vi "HistoryList.vi"(7 "Module Name":string="Module") -> ()   [LabVIEW 2017, in "DebugConsole.lvlib"]
uses:
  DebugConsole.lvlib
  508e9bfe-6490-4ffa-b47f-27ea34313f76.vi
  089f3262-7a84-4d39-9c60-bc06a6c67321.vi
  a9ada03b-0598-4474-9d19-b17bf33f6bd0.vi
  <vilib>/addons/_JKI Toolkits/State Machine/_JKI_lib_State_Machine.llb/Parse State Queue__JKI_lib_State_Machine.vi
  AdvanceAPI/CSM - Keywords.vi
  _csmlite/_Engine.vi
  _csmlite/_PassAllowedMessage - Mapping.vi
  _Polymophic/CSM - Replace Marks in Messages.vi
  <vilib>/Utility/Data Type/Get Type Information.vi
  _csmHelper/lvcsmFile/lvcsm File Path.vi
  <vilib>/Utility/config.llb/Open Config Data.vi
  <vilib>/Utility/config.llb/Write Key.vi
  <vilib>/Utility/config.llb/Write Key (Boolean).vi
  <vilib>/Utility/Data Type/Get Array Information.vi
  <vilib>/Utility/config.llb/Get Key Names.vi
  <vilib>/Utility/config.llb/Remove Key.vi
  <vilib>/Utility/config.llb/Write Key (String).vi
  _csmHelper/lvcsmFile/Path to lvcsm String.vi
  <vilib>/Utility/config.llb/Write Key (I32).vi
  <vilib>/Utility/config.llb/Write Key (Double).vi
  <vilib>/Utility/config.llb/Close Config Data.vi
  _Polymophic/Add State(s) to Queue By BOOL(Element).vi
  <vilib>/Utility/config.llb/Read Key.vi
  <vilib>/Utility/config.llb/Read Key (Boolean).vi
  <vilib>/Utility/config.llb/Read Key (String).vi
  _csmHelper/lvcsmFile/lvcsm String to Path.vi
  <vilib>/Utility/config.llb/Read Key (I32).vi
  <vilib>/Utility/config.llb/Read Key (Double).vi
  _csmHelper/lvcsmFile/_Array of VData to VCluster.vi
  _csmlite/_csmlite.lvlib
  Communicable State Machine.lvlib
  _Shared/CSM Shared.lvlib
panel:
  in  "History":i32(listbox)
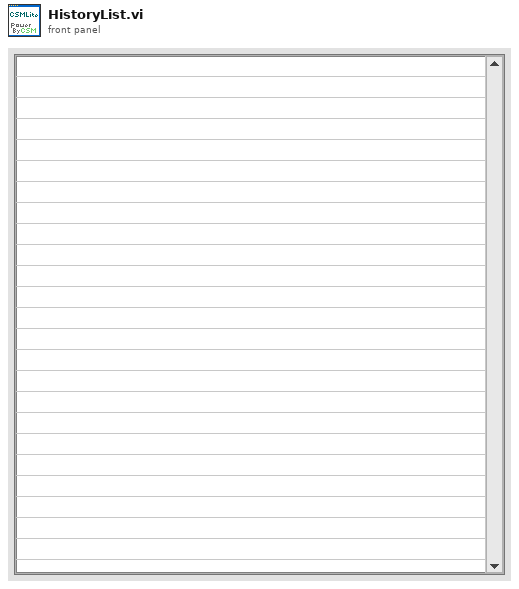
[diagram p1: front panel]
types:
  T1 = enum32{"Invalid", "Standard", "Closed", "Hidden", "Minimized", "Maximized"}
  T2 = enum32{"invalid app kind", "Development System", "Run Time System", "Student Edition", "Embedded LabVIEW", "Evaluation", "Custom"}
  T3 = cluster{"History Length":i32, "History":string[]}
  T4 = typedef "LVPoint32TypeDef.ctl" = cluster{"Horizontal":i32, "Vertical":i32}
  T5 = cluster{"Core":cluster{"Current VI Reference":refnum<vi>, "Close Panel on Exit?":bool}, "History Length":i32}
  T6 = cluster{"Current VI Reference":refnum<vi>, "Close Panel on Exit?":bool}
  T7 = cluster{"History Length":i32, "Item Names":string[]}
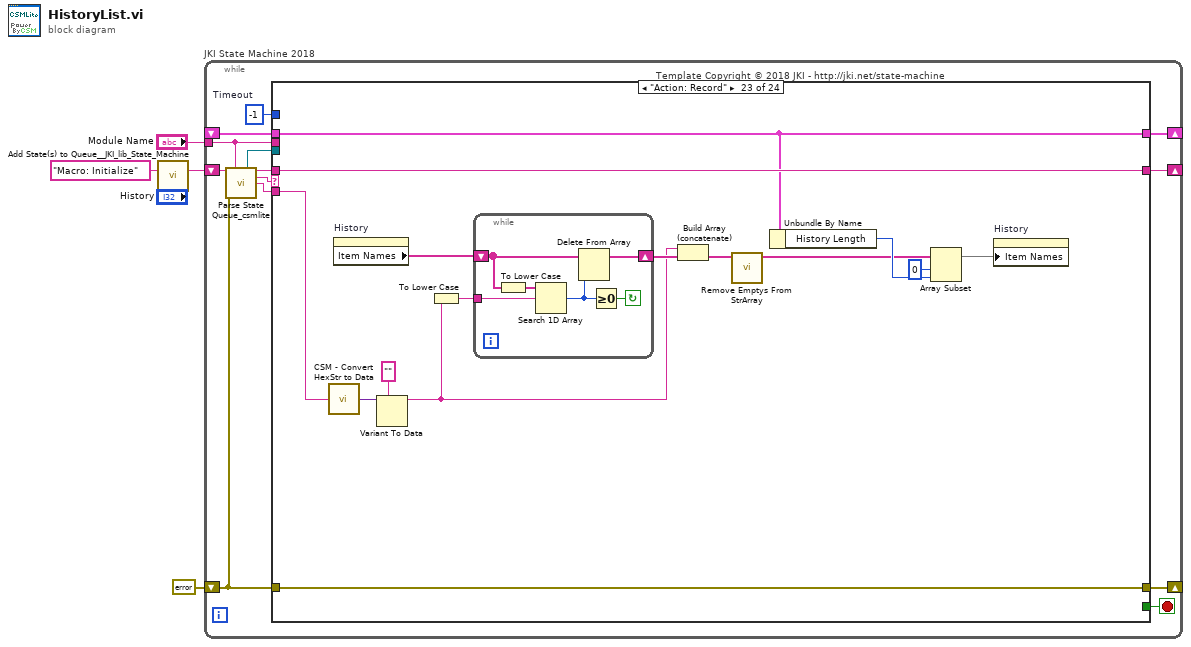
[diagram p0: block diagram]
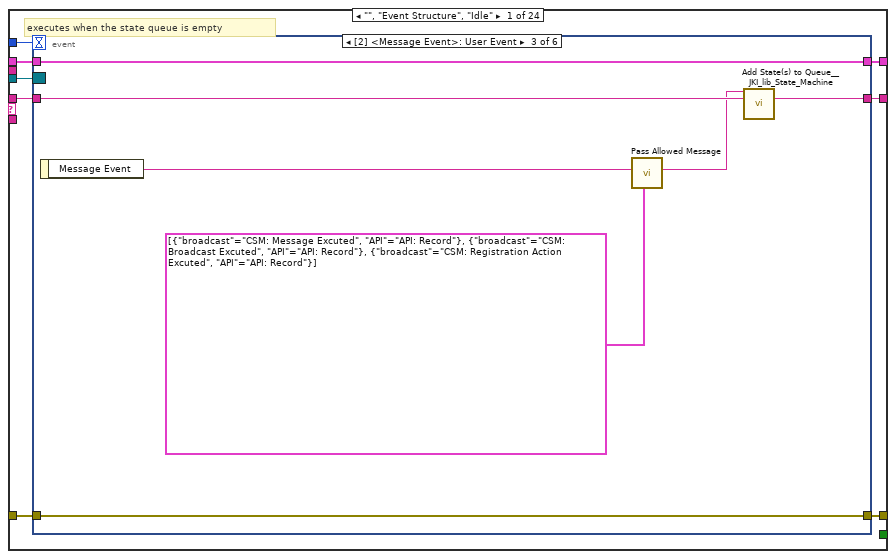
[diagram p2: hidden frame]
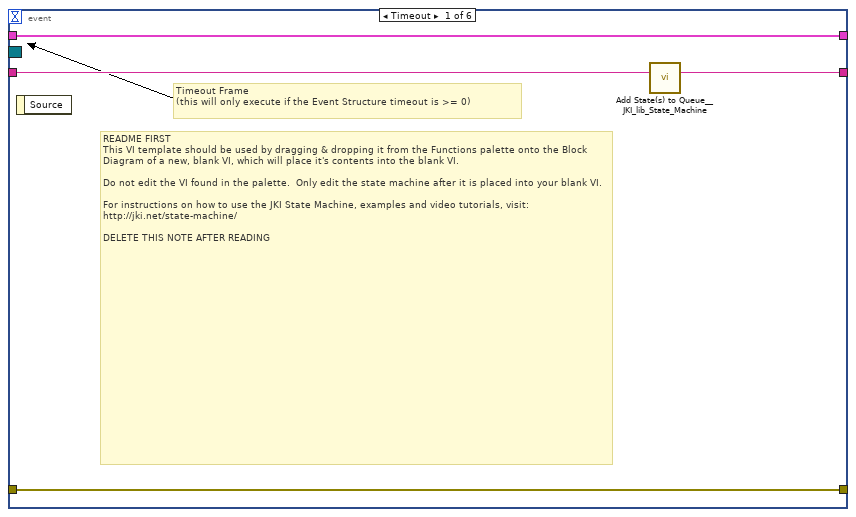
[diagram p3: hidden frame]
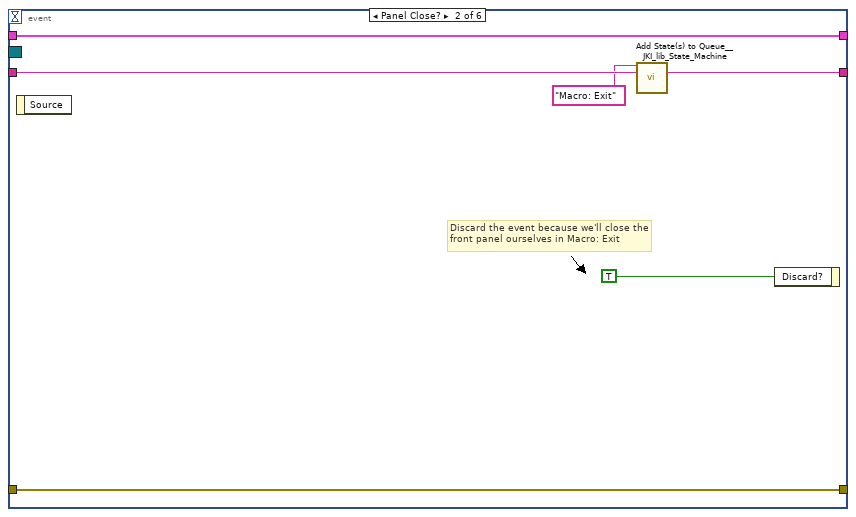
[diagram p4: hidden frame]
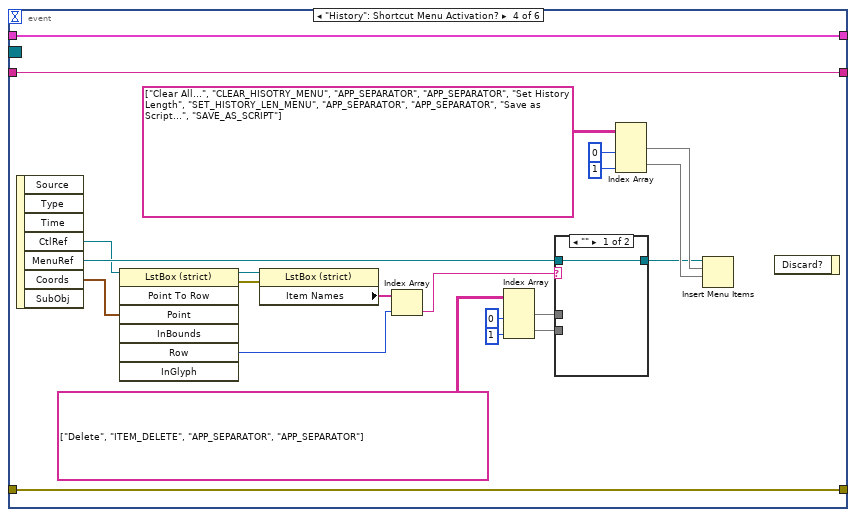
[diagram p5: hidden frame]
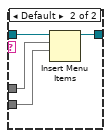
[diagram p6: hidden frame]
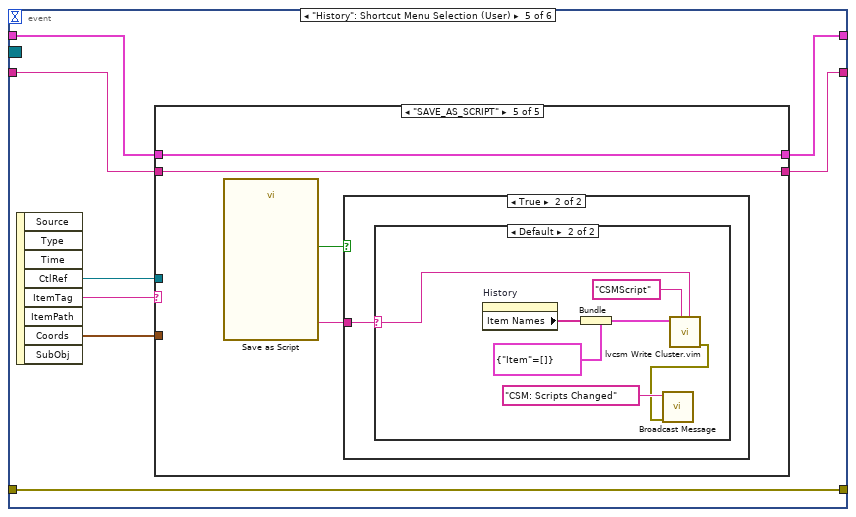
[diagram p7: hidden frame]
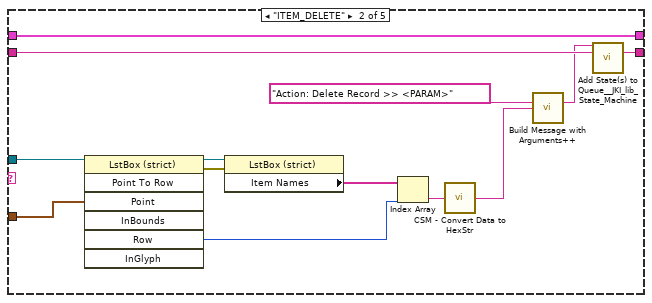
[diagram p9: hidden frame]
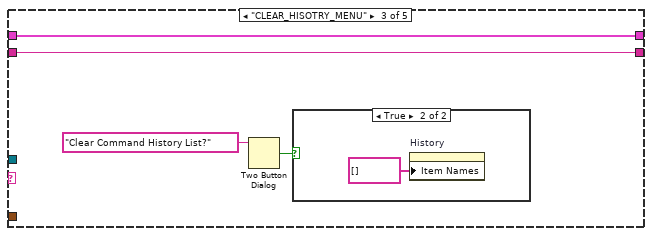
[diagram p10: hidden frame]
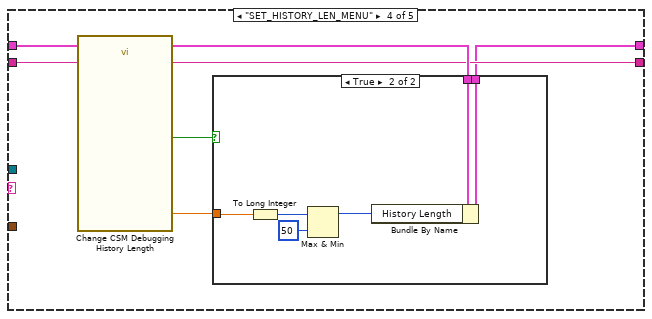
[diagram p12: hidden frame]
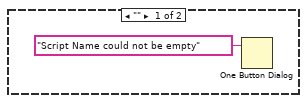
[diagram p15: hidden frame]
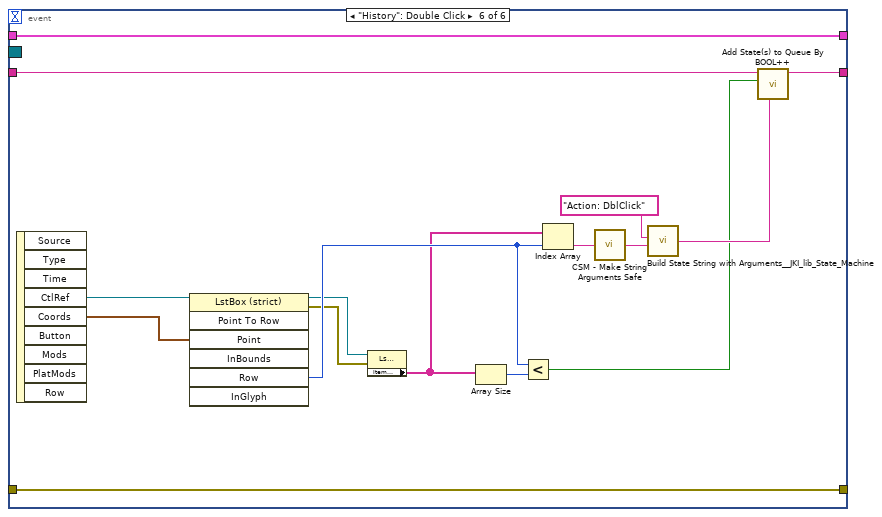
[diagram p16: hidden frame]
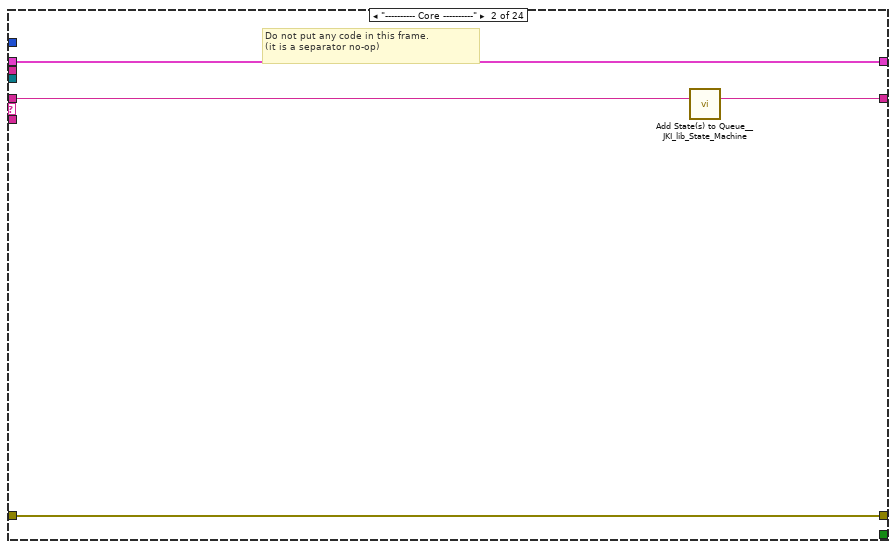
[diagram p17: hidden frame]
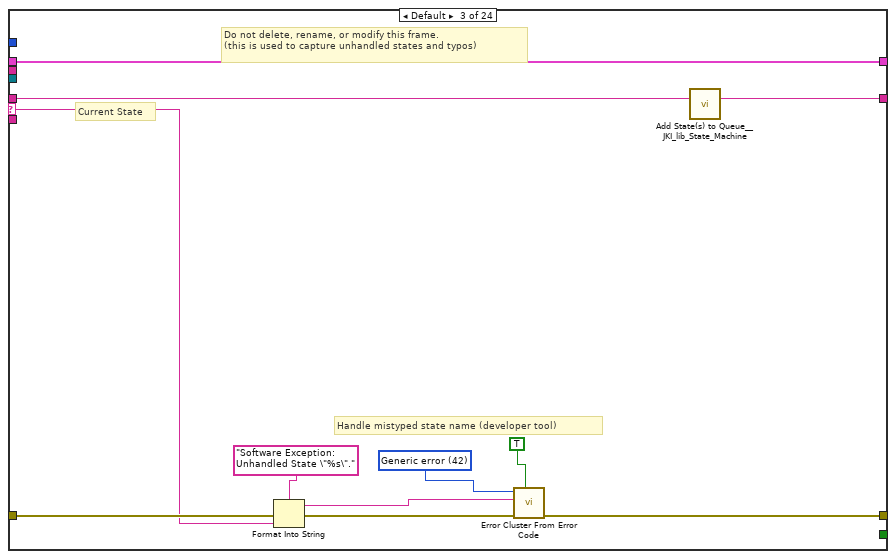
[diagram p18: hidden frame]
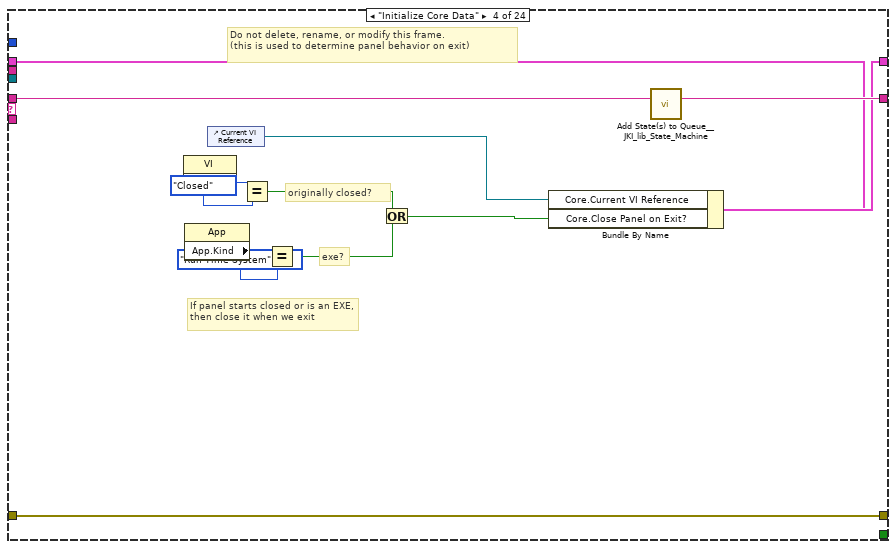
[diagram p19: hidden frame]
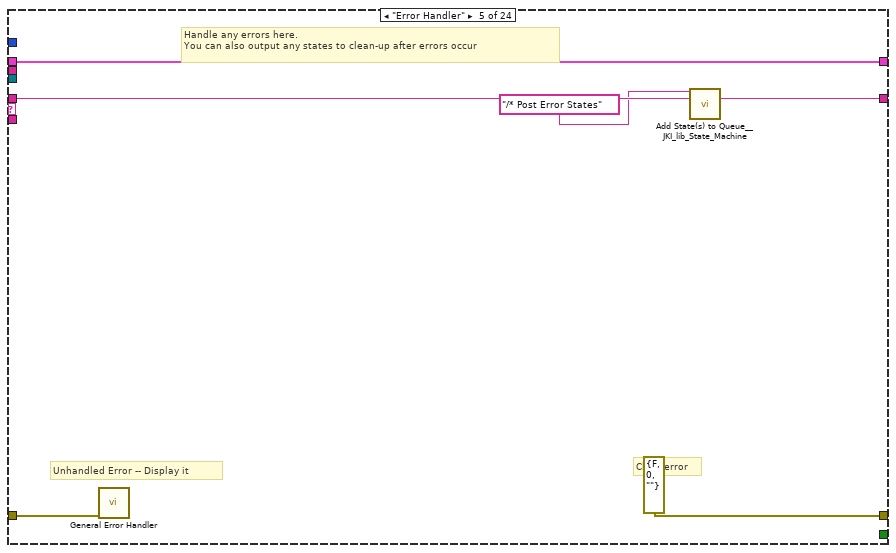
[diagram p20: hidden frame]
diagram:
  n1 = call <vilib>:"Add State(s) to Queue__JKI_lib_State_Machine.vi"("State(s) in (\"\")"="Macro: Initialize") -> ("States Out"=w3:string)  [unwired: 14 in]
  n2 = while "JKI State Machine 2018" {
    shift-right: [w10] -> _
    shift-left: _ -> [w9]
    shift-right: [w13] -> _
    shift-left: errorcluster {"status"=FALSE, "code"=0, "source"=""} ("error out") -> [w7]
    shift-right: [w12] -> _
    shift-left: w3 -> [w14]
    tunnel: "Module Name" -> [w5]
    stop <- w11 stop-if-true
    w8 = -1  # Timeout
    # "Template Copyright © 2018 JKI - http://jki.net/state-machine"
    n3 = call "Parse State Queue_csmlite.vi"("State Queue"=w14, "Current Module(\"\" to generate an ID)"=w5, "Error In (no error)"=w7) -> ("Event Registration Refnum"=w6:refnum<event-registration>, "Remaining States"=w16:string, "Current State"=w17:string, "Arguments"=w15:string)  [unwired: 9 in]
    n4 = case shown="\"Action: Record\"" w17 {
      selector: w17 -> [_ _ w143 _ _ _ _ _ _ _ _ _ _ _ _ _ _ _ _ _ _ _ _ _]
      tunnel: w16 -> [w25 w142 w147 w166 w172 w177 w181 w187 w195 w202 w209 w213 w217 w223 w234 w303 w308 w318 w320 w325 w332 w336 w350 w366]
      tunnel: w15 -> [_ _ _ _ _ _ _ _ _ _ _ _ _ w218 w228 _ _ _ _ w322 _ _ w349 w367]
      tunnel: w9 -> [w23 w139 w145 w159 w169 w175 w178 _ w194 w201 w204 w210 w215 w221 w230 w300 w305 w315 w319 w327 w329 w333 w339 w365]
      tunnel: [w22 w140 w149 w163 errorcluster {"status"=FALSE, "code"=0, "source"=""} ("error out") w174 w179 w184 w196 w203 w205 w211 w214 w219 w231 w301 w306 w316 w321 w328 w330 w334 w351 w368] -> w13
      tunnel: w7 -> [w21 w140 w148 w163 w168 w174 w179 w184 w196 w203 w206 w211 w214 w220 w232 w301 w306 w316 w321 w328 w330 w334 w351 w368]
      tunnel: [w24 w141 w146 w165 w171 w176 w180 w186 w195 w202 w208 w212 w216 w222 w233 w302 w307 w317 w320 w326 w331 w335 w350 w366] -> w12
      tunnel: [_ _ _ _ _ TRUE _ _ _ _ _ _ _ _ _ _ _ _ _ _ _ _ _ _] -> w11
      tunnel: [w20 w139 w145 w164 w169 w175 w178 w185 w191 w201 w204 w210 w215 w221 w230 w300 w305 w315 w319 w327 w329 w333 w339 w365] -> w10
      tunnel: w8 -> [w19 _ _ _ _ _ _ _ _ _ _ _ _ _ _ _ _ _ _ _ _ _ _ _]
      tunnel: w6 -> [w18 _ _ _ _ _ _ _ _ _ _ _ _ _ _ _ _ _ _ _ _ _ _ _]
      tunnel: w5 -> [_ _ _ _ _ _ _ _ w189 w198 _ _ _ _ _ _ _ _ _ _ _ _ _ _]
      frame "", "Event Structure", "Idle" {
        # "executes when the state queue is empty"
        n5 = event shown="[2] <Message Event>: User Event" {
          selector: w18 -> [_ _ _ _ _ _]
          dyn-events: _ -> [_ _ _ _ _ _]
          timeout: w19 -> [_ _ _ _ _ _]
          tunnel: w25 -> [w29 w35 w40 w64 w73 w138]
          tunnel: [w28 w34 w38 w64 w72 w125] -> w24
          tunnel: w23 -> [w26 w32 w41 w62 w76 w136]
          tunnel: [w27 w33 w42 w63 w77 w137] -> w22
          tunnel: w21 -> [w27 w33 w42 w63 w77 w137]
          tunnel: [w26 w32 w41 w62 w75 w136] -> w20
          event Timeout {
            # "README FIRST\nThis VI template should be used by dragging & dropping it from the Functions palette onto the Block Diagram of a new, blank VI, which will place it's contents into the blank VI.\n\nDo not edit the VI found in the palette.  Only edit the state machine after it is placed into your blank VI.\n\nFor instructions on how to use the JKI State Machine, examples and video tutorials, visit:\nhttp://jki.net/state-machine/\n\nDELETE THIS NOTE AFTER READING"
            # "Timeout Frame\n(this will only execute if the Event Structure timeout is >= 0)"
            n6 = event-data() -> ()  [unwired: 1 in, 1 out]
            n7 = call <vilib>:"Add State(s) to Queue__JKI_lib_State_Machine.vi"("State(s) in (\"\")"=w29) -> ("States Out"=w28:string)  [unwired: 14 in]
          }
          event Panel Close? {
            # "Discard the event because we'll close the front panel ourselves in Macro: Exit"
            n8 = event-data() -> ()  [unwired: 1 in, 1 out]
            n9 = call <vilib>:"Add State(s) to Queue__JKI_lib_State_Machine.vi"("State(s) in Front (\"\")"="Macro: Exit", "State(s) in (\"\")"=w35) -> ("States Out"=w34:string)  [unwired: 13 in]
            n10 = event-data("Discard?"=TRUE) -> ()  [unwired: 1 in, 1 out]
          }
          event User Event {
            n11 = event-data() -> ("Message Event"=w39:string)  [unwired: 1 in]
            n12 = call-poly "Pass Allowed Message.vi"("Mapping"=cluster{"broadcast":string, "API":string}[] [{"broadcast"="CSM: Message Excuted", "API"="API: Record"}, {"broadcast"="CSM: Broadcast Excuted", "API"="API: Record"}, {"broadcast"="CSM: Registration Action Excuted", "API"="API: Record"}], "JKISM External Event"=w39) -> ("States"=w37:string)  [unwired: 7 in]
            n13 = call <vilib>:"Add State(s) to Queue__JKI_lib_State_Machine.vi"("State(s) in Front (\"\")"=w37, "State(s) in (\"\")"=w40) -> ("States Out"=w38:string)  [unwired: 13 in]
          }
          event "History": Shortcut Menu Activation? {
            n14 = event-data() -> ("CtlRef"=w46:refnum<vi>, "MenuRef"=w54:refnum<k9>, "Coords"=w45:T4)  [unwired: 1 in, 4 out]
            n15 = invoke class="LstBox (strict)" method="Point To Row"(reference=w46, "Point"=w45) -> (reference out=w47:refnum<vi>, error out=w43:errorcluster, "Row"=w44:i32)  [unwired: 5 in, 4 out]
            n16 = property class="LstBox (strict)"(reference=w47, error in=w43) -> ("Item Names"=w56:string[])  [unwired: 2 out]
            n17 = Index Array(array=w56, index=w44) -> (element=w48:string)
            n18 = Index Array(array=string[][] [["Delete", "ITEM_DELETE"], ["APP_SEPARATOR", "APP_SEPARATOR"]] ("item names"), index (col) #1=0 ("index (row)"), index (col) #2=1 ("index (row)")) -> (element #1=w51:string[], element #2=w49:string[])  [unwired: 2 in]
            n19 = case shown="\"\"" w48 {
              tunnel: [w65 w69] -> w55
              tunnel: w54 -> [w65 w68]
              tunnel: w51 -> [_ w67]
              tunnel: w49 -> [_ w66]
              frame "" {
              }
              frame Default {
                n20 = Insert Menu Items(7:w66, 8:w67, 9:w68) -> (3:w69:refnum<k9>)  [unwired: 3 in, 2 out]
              }
            }
            n21 = Index Array(array=string[][] [["Clear All...", "CLEAR_HISOTRY_MENU"], ["APP_SEPARATOR", "APP_SEPARATOR"], ["Set History Length", "SET_HISTORY_LEN_MENU"], ["APP_SEPARATOR", "APP_SEPARATOR"], ["Save as Script...", "SAVE_AS_SCRIPT"]] ("item names"), index (col) #1=0 ("index (row)"), index (col) #2=1 ("index (row)")) -> (element #1=w60:string[], element #2=w59:string[])  [unwired: 2 in]
            n22 = Insert Menu Items(7:w59, 8:w60, 9:w55) -> ()  [unwired: 3 in, 3 out]
            n23 = event-data() -> ()  [unwired: 2 in, 1 out]
          }
          event "History": Shortcut Menu Selection (User) {
            n24 = event-data() -> ("CtlRef"=w71:refnum<vi>, "ItemTag"=w74:string, "Coords"=w70:T4)  [unwired: 1 in, 5 out]
            n25 = case shown="\"SAVE_AS_SCRIPT\"" w74 {
              tunnel: w76 -> [w79 w92 w93 w102 w110]
              tunnel: [w78 w91 w95 w101 w113] -> w72
              tunnel: [w79 w92 w93 w100 w110] -> w75
              tunnel: w73 -> [w78 w90 w95 w101 w113]
              tunnel: w71 -> [_ w83 _ _ _]
              tunnel: w70 -> [_ w81 _ _ _]
              frame Default {
              }
              frame "ITEM_DELETE" {
                n26 = invoke class="LstBox (strict)" method="Point To Row"(reference=w83, "Point"=w81) -> (reference out=w85:refnum<vi>, error out=w84:errorcluster, "Row"=w80:i32)  [unwired: 5 in, 4 out]
                n27 = property class="LstBox (strict)"(reference=w85, error in=w84) -> ("Item Names"=w82:string[])  [unwired: 2 out]
                n28 = Index Array(array=w82, index=w80) -> (element=w87:string)
                n29 = call "CSM - Convert Data to HexStr.vi"("Variant"=w87) -> ("HEX String (0-9,A-F)"=w86:string)  [unwired: 8 in]
                n30 = call-poly "Build Message with Arguments++.vi"("States With Replace Token"="Action: Delete Record >> <PARAM>" ("State(s) in Front (\"\")"), "<param>"=w86) -> ("States"=w89:string)  [unwired: 13 in]
                n31 = call <vilib>:"Add State(s) to Queue__JKI_lib_State_Machine.vi"("State(s) in Front (\"\")"=w89, "State(s) in (\"\")"=w90) -> ("States Out"=w91:string)  [unwired: 13 in]
              }
              frame "CLEAR_HISOTRY_MENU" {
                n32 = Two Button Dialog(message="Clear Command History List?") -> (T button?=w94:bool)  [unwired: 2 in]
                n33 = case shown="True" w94 {
                  frame False {
                  }
                  frame True {
                    n34 = property on="History" class="LstBox (strict)"("Item Names"=string[] []) -> ()  [unwired: 2 in, 2 out]
                  }
                }
              }
              frame "SET_HISTORY_LEN_MENU" {
                n35 = call "Change CSM Debugging History Length"() -> ("History Length"=w99:dbl, "OK"=w98:bool)  [unwired: 17 in, 1 out]
                n36 = case shown="True" w98 {
                  tunnel: w102 -> [w103 w109]
                  tunnel: [w103 w108] -> w100
                  tunnel: w99 -> [_ w106]
                  frame False {
                  }
                  frame True {
                    n37 = To Long Integer(number=w106) -> (32bit integer=w104:i32)
                    n38 = Max & Min(x=w104, y=50) -> (max(x,y)=w107:i32)  [unwired: 1 out]
                    n39 = Bundle By Name(cluster=w109, "History Length"=w107) -> (w108:T5)
                  }
                }
              }
              frame "SAVE_AS_SCRIPT" {
                n40 = call "Save as Script"() -> ("Script"=w112:string, "OK"=w111:bool)  [unwired: 17 in, 1 out]
                n41 = case shown="True" w111 {
                  tunnel: w112 -> [_ w114]
                  frame False {
                  }
                  frame True {
                    n42 = case shown="Default" w114 {
                      selector: w114 -> [_ w121]
                      frame "" {
                        n43 = One Button Dialog(message="Script Name could not be empty") -> ()  [unwired: 1 in, 1 out]
                      }
                      frame Default {
                        n44 = property on="History" class="LstBox (strict)"() -> ("Item Names"=w120:string[])  [unwired: 2 in, 2 out]
                        n45 = Bundle(cluster=cluster{"Item":string[]} {"Item"=[]}, "Item"=w120) -> (w119:cluster{"Item":string[]})
                        n46 = call "lvcsm Write Cluster.vim"("Sub-section (\"\")"=w121, "Section"="CSMScript", "Configuration"=w119) -> ("error out"=w116:errorcluster)  [unwired: 8 in]
                        n47 = call "Broadcast Message.vi"("Error in"=w116, "Message"="CSM: Scripts Changed") -> ()  [unwired: 9 in, 1 out]
                      }
                    }
                  }
                }
              }
            }
          }
          event "History": Double Click {
            n48 = event-data() -> ("CtlRef"=w127:refnum<vi>, "Coords"=w126:T4)  [unwired: 1 in, 7 out]
            n49 = invoke class="LstBox (strict)" method="Point To Row"(reference=w127, "Point"=w126) -> (reference out=w129:refnum<vi>, error out=w130:errorcluster, "Row"=w135:i32)  [unwired: 5 in, 4 out]
            n50 = property class="LstBox (strict)"(reference=w129, error in=w130) -> ("Item Names"=w132:string[])  [unwired: 2 out]
            n51 = Array Size(array=w132) -> (size(s)=w131:i32)
            n52 = Less?(x=w135, y=w131) -> (x < y?=w123:bool)
            n53 = Index Array(array=w132, index=w135) -> (element=w133:string)
            n54 = call "CSM - Make String Arguments Safe.vi"("Argument String"=w133) -> ("Safe Argument String"=w134:string)  [unwired: 8 in]
            n55 = call <vilib>:"Build State String with Arguments__JKI_lib_State_Machine.vi"("Arguments (\"\")"=w134, "State"="Action: DblClick") -> ("State with Arguments"=w124:string)  [unwired: 4 in]
            n56 = call-poly "Add State(s) to Queue By BOOL++.vi"("TRUE (\"\")"=w124, "Condition"=w123, "State Queue (\"\")"=w138) -> ("Remaining States"=w125:string)  [unwired: 8 in]
          }
        }
      }
      frame "---------- Core ----------" {
        # "Do not put any code in this frame.\n(it is a separator no-op)"
        n57 = call <vilib>:"Add State(s) to Queue__JKI_lib_State_Machine.vi"("State(s) in (\"\")"=w142) -> ("States Out"=w141:string)  [unwired: 14 in]
      }
      frame Default {
        w152 = 42 items=["No error", "Argument error", "Memory is full", "Out of zone", "End of file", "File already open", "Generic file I/O error", "File not found", "File permission error", "Disk is full", "Duplicate path", "Too many files open", "System feature not enabled", "Resource file not found", "Cannot add resource", "Resource not found", "Image not found", "Image memory error", "Pen does not exist", "Config type invalid", "Config token not found", "Config parse error", "Config memory error", "Bad external code format", "Bad external code offset", "External code not present", "Null window", "Destroy window error", "Null menu", "Print aborted", "Bad print record", "Print driver error", "Windows error during printing", "Memory error during printing", "Print dialog error", "Generic print error", "Invalid device refnum", "Device not found", "Device parameter error", "Device unit error", "Cannot open device", "Device call aborted", "Generic error", "Cancelled by user", "Object ID too low", "Object ID too high", "Object not in heap", "Unknown heap", "Unknown object (invalid DefProc)", "Unknown object (DefProc not in table)", "Message out of range", "Invalid (null) method", "Unknown message", "Manager call not supported", "Bad address", "Network operation in progress", "Network operation timed out", "Connection is busy", "Network attribute not supported", "Network error", "Address in use", "System out of memory", "Connection aborted", "Connection refused", "Not connected", "Already connected", "Connection closed", "Initialization error (interapplication manager)", "Bad occurrence", "Wait on unbound occurrence handler", "Occurrence queue overflow", "Datalog type conflict", "Unused", "Unrecognized type (interapplication manager)", "Memory corrupt", "Failed to make temporary DLL", "Old CIN version", "Drag socket not found", "Failed to load drop-object", "Failed to register OLE object", "Failed to release OLE object", "Format specifier type mismatch", "Unknown format specifier", "Too few format specifiers", "Too many format specifiers", "Scan failed", "Newer CIN version", "Error converting to variant", "Runtime menu error", "Password tampered", "Variant attribute not found", "Incompatible variant data type", "Event data is not available", "Event Store is not present", "Occurrence is not found", "Event Queue is not created", "Event info is not available", "Refnum passed is NULL", "Error retrieving Class GUID", "Error retrieving CoClass GUID", "Error retrieving TypeLib GUID.", "Bad built application magic bytes.", "Specific driver is different from the specific driver associated with the Logical Name.", "There is no session opened to the class driver.", "Max Error", "MAX - Error with config objects", "MAX - Error loading configuration", "MAX - Group not supported"]
        # "Current State"
        # "Do not delete, rename, or modify this frame.\n(this is used to capture unhandled states and typos)"
        # "Handle mistyped state name (developer tool)"
        n58 = Format Into String(format string="Software Exception: Unhandled State \"%s\"." ("message"), error in=w148, w143) -> (resulting string=w151:string, error out=w150:errorcluster)  [unwired: 1 in]
        n59 = call <vilib>:"Error Cluster From Error Code.vi"("show call chain? (False)"=TRUE, "error in (no error)"=w150, "error message (\"\")"=w151, "error code (0)"=w152) -> ("error out"=w149:errorcluster)  [unwired: 5 in]
        n60 = call <vilib>:"Add State(s) to Queue__JKI_lib_State_Machine.vi"("State(s) in (\"\")"=w147) -> ("States Out"=w146:string)  [unwired: 14 in]
      }
      frame "Initialize Core Data" {
        # "Do not delete, rename, or modify this frame.\n(this is used to determine panel behavior on exit)"
        # "originally closed?"
        # "exe?"
        # "If panel starts closed or is an EXE, then close it when we exit"
        n61 = property class="VI"() -> ("FP.State"=w156:T1)  [unwired: 2 in, 2 out]
        n62 = property class="App"() -> ("App.Kind"=w162:T2)  [unwired: 2 in, 2 out]
        n63 = control-ref of="Current VI Reference"() -> (w157:refnum<vi>)
        n64 = Equal?(x=w156, y=T1."Closed" ("Front Panel Window:State")) -> (x = y?=w154:bool)
        n65 = Equal?(x=w162, y=T2."Run Time System" ("Application:Kind")) -> (x = y?=w160:bool)
        n66 = Or(x=w154, y=w160) -> (x .or. y?=w158:bool)
        n67 = Bundle By Name(cluster=w159, "Core.Current VI Reference"=w157, "Core.Close Panel on Exit?"=w158) -> (w164:T5)
        n68 = call <vilib>:"Add State(s) to Queue__JKI_lib_State_Machine.vi"("State(s) in (\"\")"=w166) -> ("States Out"=w165:string)  [unwired: 14 in]
      }
      frame "Error Handler" {
        # "Unhandled Error -- Display it"
        # "Handle any errors here.\nYou can also output any states to clean-up after errors occur"
        # "Clear error"
        n69 = call <vilib>:"General Error Handler.vi"("error in (no error)"=w168) -> ()  [unwired: 10 in, 5 out]
        n70 = call <vilib>:"Add State(s) to Queue__JKI_lib_State_Machine.vi"("State(s) in Front (\"\")"="/* Post Error States", "State(s) in (\"\")"=w172) -> ("States Out"=w171:string)  [unwired: 13 in]
      }
      frame "Exit" {
        # "Do not put any code in this frame.\n(No errors that occur here will be handled.)"
        n71 = call <vilib>:"Add State(s) to Queue__JKI_lib_State_Machine.vi"("State(s) in (\"\")"=w177) -> ("States Out"=w176:string)  [unwired: 14 in]
      }
      frame "---------- Data ----------" {
        # "Do not put any code in this frame.\n(It is a separator no-op. You can make a copy of this frame to create a new Data frame)"
        n72 = call <vilib>:"Add State(s) to Queue__JKI_lib_State_Machine.vi"("State(s) in (\"\")"=w181) -> ("States Out"=w180:string)  [unwired: 14 in]
      }
      frame "Data: Initialize" {
        w182 = 50  # History Length
        w183 = T6 {"Current VI Reference"=refnum, "Close Panel on Exit?"=FALSE}  # Core
        n73 = Bundle("Core"=w183, "History Length"=w182) -> (w185:T5)  [unwired: 1 in]
        n74 = call <vilib>:"Add State(s) to Queue__JKI_lib_State_Machine.vi"("State(s) in (\"\")"=w187) -> ("States Out"=w186:string)  [unwired: 14 in]
      }
      frame "Data: Load Configuration" {
        n75 = call "lvcsm Read Cluster.vim"("Section"=w189, "Default Prototype"=T3 {"History Length"=50, "History"=[]}) -> ("Cluster (Dup)"=w193:T3)  [unwired: 8 in, 1 out]
        n76 = Unbundle By Name(w193) -> ("History Length"=w190:i32, "History"=w188:string[])
        n77 = Bundle By Name(cluster=w194, "History Length"=w190) -> (w191:T5)
        n78 = property on="History" class="LstBox (strict)"("Item Names"=w188) -> ()  [unwired: 2 in, 2 out]
      }
      frame "Data: Save Configuration" {
        n79 = Unbundle By Name(w201) -> ("History Length"=w200:i32)
        n80 = property on="History" class="LstBox (strict)"() -> ("Item Names"=w197:string[])  [unwired: 2 in, 2 out]
        n81 = Bundle("History Length"=w200, "Item Names"=w197) -> (w199:T7)  [unwired: 1 in]
        n82 = call "lvcsm Write Cluster.vim"("Section"=w198, "Configuration"=w199) -> ()  [unwired: 9 in, 1 out]
      }
      frame "Data: Cleanup" {
        # "Cleanup any data and references, here.\n(this is called automatically, by the Macro: Exit)"
        n83 = Unbundle By Name(w204) -> ("Core.Current VI Reference"=w207:refnum<vi>)
        n84 = Close Reference(reference=w207, error in (no error)=w206) -> (error out=w205:errorcluster)
        n85 = call <vilib>:"Add State(s) to Queue__JKI_lib_State_Machine.vi"("State(s) in (\"\")"=w209) -> ("States Out"=w208:string)  [unwired: 14 in]
      }
      frame "---------- UI ----------" {
        # "Do not put any code in this frame.\n(It is a separator no-op. You can make a copy of this frame to create a new UI frame)"
        n86 = call <vilib>:"Add State(s) to Queue__JKI_lib_State_Machine.vi"("State(s) in (\"\")"=w213) -> ("States Out"=w212:string)  [unwired: 14 in]
      }
      frame "UI: Initialize" {
        # "Initialize the User Interface, here.\n(this is called automatically, by the Macro: Init)"
        n87 = call <vilib>:"Add State(s) to Queue__JKI_lib_State_Machine.vi"("State(s) in (\"\")"=w217) -> ("States Out"=w216:string)  [unwired: 14 in]
      }
      frame "UI: Cursor Set" {
        # "Argument"
        # "Set and Unset Cursor Busy.\n(Usage: \"UI: Cursor Set >> Busy|Idle\")"
        n88 = case shown="\"Idle\", Default" w218 {
          tunnel: w220 -> [w225 w227]
          tunnel: [w224 w226] -> w219
          frame "Idle", Default {
            n89 = call <vilib>:"Unset Busy.vi"("error in (no error)"=w225) -> ("error out"=w224:errorcluster)  [unwired: 10 in]
          }
          frame "Busy" {
            n90 = call <vilib>:"Set Busy.vi"("error in (no error)"=w227) -> ("error out"=w226:errorcluster)  [unwired: 9 in, 1 out]
          }
        }
        n91 = call <vilib>:"Add State(s) to Queue__JKI_lib_State_Machine.vi"("State(s) in (\"\")"=w223) -> ("States Out"=w222:string)  [unwired: 14 in]
      }
      frame "UI: Front Panel State" {
        # "Argument"
        # "Set Front Panel Open or Closed\n(Usage: \"UI: Front Panel State >> Open|Close\")"
        n92 = Unbundle By Name(w230) -> ("Core.Current VI Reference"=w229:refnum<vi>)
        n93 = case shown="\"Minimize\", \"Minimized\"" w228 {
          tunnel: w232 -> [w240 w255 w266 w279 w292]
          tunnel: [w242 w256 w268 w281 w294] -> w231
          tunnel: w229 -> [w241 w253 w267 w280 w293]
          frame "Open", "Standard", Default {
            w235 = T1."Standard" ("State")
            n94 = property class="VI"(reference=w241, error in=w240) -> (reference out=w238:refnum<vi>, error out=w239:errorcluster, "FP.State"=w237:T1)
            n95 = Not Equal?(x=w237, y=w235) -> (x != y?=w236:bool)
            n96 = case shown="True" w236 {
              tunnel: [w246 w248] -> w242
              tunnel: w239 -> [w245 w248]
              tunnel: w238 -> [w244 _]
              tunnel: w235 -> [w243 _]
              frame True {
                n97 = invoke class="VI" method="FP.Open"(reference=w244, error in=w245, "Activate"=TRUE, "State"=w243) -> (error out=w246:errorcluster)  [unwired: 1 in, 4 out]
              }
              frame False {
              }
            }
          }
          frame "Close", "Closed" {
            n98 = property class="VI"(reference=w253, error in=w255) -> (reference out=w252:refnum<vi>, error out=w254:errorcluster, "FP.State"=w250:T1)
            n99 = Not Equal?(x=w250, y=T1."Closed" ("Front Panel Window:State")) -> (x != y?=w249:bool)
            n100 = case shown="True" w249 {
              tunnel: [w257 w260] -> w256
              tunnel: w254 -> [w257 w259]
              tunnel: w252 -> [_ w258]
              frame False {
              }
              frame True {
                n101 = invoke class="VI" method="FP.Close"(reference=w258, error in=w259) -> (error out=w260:errorcluster)  [unwired: 1 in, 2 out]
              }
            }
          }
          frame "Hidden", "Hide" {
            w261 = T1."Hidden" ("State")
            n102 = property class="VI"(reference=w267, error in=w266) -> (reference out=w264:refnum<vi>, error out=w265:errorcluster, "FP.State"=w263:T1)
            n103 = Not Equal?(x=w263, y=w261) -> (x != y?=w262:bool)
            n104 = case shown="True" w262 {
              tunnel: [w272 w273] -> w268
              tunnel: w265 -> [w271 w273]
              tunnel: w264 -> [w270 _]
              tunnel: w261 -> [w269 _]
              frame True {
                n105 = invoke class="VI" method="FP.Open"(reference=w270, error in=w271, "State"=w269) -> (error out=w272:errorcluster)  [unwired: 2 in, 4 out]
              }
              frame False {
              }
            }
          }
          frame "Minimize", "Minimized" {
            w274 = T1."Minimized" ("State")
            n106 = property class="VI"(reference=w280, error in=w279) -> (reference out=w277:refnum<vi>, error out=w278:errorcluster, "FP.State"=w276:T1)
            n107 = Not Equal?(x=w276, y=w274) -> (x != y?=w275:bool)
            n108 = case shown="True" w275 {
              tunnel: [w285 w286] -> w281
              tunnel: w278 -> [w284 w286]
              tunnel: w277 -> [w283 _]
              tunnel: w274 -> [w282 _]
              frame True {
                n109 = invoke class="VI" method="FP.Open"(reference=w283, error in=w284, "State"=w282) -> (error out=w285:errorcluster)  [unwired: 2 in, 4 out]
              }
              frame False {
              }
            }
          }
          frame "Maximize", "Maximized" {
            w287 = T1."Maximized" ("State")
            n110 = property class="VI"(reference=w293, error in=w292) -> (reference out=w290:refnum<vi>, error out=w291:errorcluster, "FP.State"=w289:T1)
            n111 = Not Equal?(x=w289, y=w287) -> (x != y?=w288:bool)
            n112 = case shown="True" w288 {
              tunnel: [w298 w299] -> w294
              tunnel: w291 -> [w297 w299]
              tunnel: w290 -> [w296 _]
              tunnel: w287 -> [w295 _]
              frame True {
                n113 = invoke class="VI" method="FP.Open"(reference=w296, error in=w297, "State"=w295) -> (error out=w298:errorcluster)  [unwired: 2 in, 4 out]
              }
              frame False {
              }
            }
          }
        }
        n114 = call <vilib>:"Add State(s) to Queue__JKI_lib_State_Machine.vi"("State(s) in (\"\")"=w234) -> ("States Out"=w233:string)  [unwired: 14 in]
      }
      frame "---------- Macro ----------" {
        # "Do not put any code in this frame.\n(It is a separator no-op. You can make a copy of this frame to create a new Macro frame)"
        n115 = call <vilib>:"Add State(s) to Queue__JKI_lib_State_Machine.vi"("State(s) in (\"\")"=w303) -> ("States Out"=w302:string)  [unwired: 14 in]
      }
      frame "Macro: Initialize" {
        # "Initialization Macro\n(This is called once, when the VI starts)"
        n116 = call <vilib>:"Add State(s) to Queue__JKI_lib_State_Machine.vi"("State(s) in Front (\"\")"="Data: Initialize\nInitialize Core Data\nData: Load Configuration\nUI: Initialize\n// UI: Front Panel State >> Open", "State(s) in (\"\")"=w308) -> ("States Out"=w307:string)  [unwired: 13 in]
      }
      frame "Macro: Exit" {
        # "Exit Macro\n(This is called once, when the VI exits)"
        n117 = Unbundle By Name(w315) -> ("Core.Close Panel on Exit?"=w314:bool)
        n118 = Select(t="UI: Front Panel State >> Close", s=w314, f="") -> (s? t:f=w311:string)
        n119 = call <vilib>:"Add State(s) to Queue__JKI_lib_State_Machine.vi"("State(s) in (\"\")"=w311, "State(s) at Back (\"\")"="Data: Save Configuration\nData: Cleanup\nExit") -> ("States Out"=w309:string)  [unwired: 13 in]
        n120 = call <vilib>:"Add State(s) to Queue__JKI_lib_State_Machine.vi"("State(s) in Front (\"\")"=w309, "State(s) in (\"\")"=w318) -> ("States Out"=w317:string)  [unwired: 13 in]
      }
      frame "------------- API ---------------" {
      }
      frame "API: Record" {
        n121 = call-poly "Build Message with Arguments++.vi"("States With Replace Token"="Action: Record >> <param>" ("State(s) in Front (\"\")"), "<param>"=w322) -> ("States"=w324:string)  [unwired: 13 in]
        n122 = call <vilib>:"Add State(s) to Queue__jki_lib_state_machine.vi"("State(s) in Front (\"\")"=w324, "State(s) in (\"\")"=w325) -> ("States Out"=w326:string)  [unwired: 13 in]
      }
      frame "---------- New Category ----------" {
        # "Template Separator\n(You can make a copy of, or modify, this frame)"
        n123 = call <vilib>:"Add State(s) to Queue__JKI_lib_State_Machine.vi"("State(s) in (\"\")"=w332) -> ("States Out"=w331:string)  [unwired: 14 in]
      }
      frame "Action: DblClick" {
        # "Your code here.\n(You can make a copy of, or modify, this frame)"
        n124 = call <vilib>:"Add State(s) to Queue__JKI_lib_State_Machine.vi"("State(s) in (\"\")"=w336) -> ("States Out"=w335:string)  [unwired: 14 in]
      }
      frame "Action: Record" {
        n125 = call "CSM - Convert HexStr to Data.vi"("HEX String"=w349) -> ("Variant"=w347:variant)  [unwired: 7 in, 1 out]
        n126 = property on="History" class="LstBox (strict)"() -> ("Item Names"=w342:string[])  [unwired: 2 in, 2 out]
        n127 = Variant To Data(type="", Variant=w347) -> (data=w344:string)  [unwired: 1 in, 1 out]
        n128 = To Lower Case(string=w344) -> (all lower case string=w343:string)
        n129 = while {
          tunnel: w343 -> [w352]
          shift-right: [w355] -> w345
          shift-left: w342 -> [w356]
          stop <- w353 continue-if-true
          n130 = To Lower Case(string=w356) -> (all lower case string=w357:string[])
          n131 = Search 1D Array(1D array=w357, element=w352) -> (index of element=w354:i32)  [unwired: 1 in]
          n132 = Delete From Array(array=w356, index=w354) -> (array with subset deleted=w355:string[])  [unwired: 1 in, 1 out]
          n133 = Greater Or Equal To 0?(x=w354) -> (x >= 0?=w353:bool)
        }
        n134 = Build Array (concatenate)(w344, w345) -> (w348:string[])
        n135 = call "Remove Emptys From StrArray.vi"("Array In"=w348) -> ("Array Out"=w338:string[])  [unwired: 10 in]
        n136 = Unbundle By Name(w339) -> ("History Length"=w341:i32)
        n137 = Array Subset(array=w338, index=0, length=w341) -> (w337:string[])
        n138 = property on="History" class="LstBox (strict)"("Item Names"=w337) -> ()  [unwired: 2 in, 2 out]
      }
      frame "Action: Delete Record" {
        n139 = property on="History" class="LstBox (strict)"() -> ("Item Names"=w359:string[])  [unwired: 2 in, 2 out]
        n140 = call "CSM - Convert HexStr to Data.vi"("HEX String"=w367) -> ("Variant"=w364:variant)  [unwired: 7 in, 1 out]
        n141 = Variant To Data(type="", Variant=w364) -> (data=w361:string)  [unwired: 1 in, 1 out]
        n142 = To Lower Case(string=w361) -> (all lower case string=w360:string)
        n143 = while {
          tunnel: w360 -> [w369]
          shift-right: [w372] -> w362
          shift-left: w359 -> [w373]
          stop <- w370 continue-if-true
          n144 = To Lower Case(string=w373) -> (all lower case string=w374:string[])
          n145 = Search 1D Array(1D array=w374, element=w369) -> (index of element=w371:i32)  [unwired: 1 in]
          n146 = Delete From Array(array=w373, index=w371) -> (array with subset deleted=w372:string[])  [unwired: 1 in, 1 out]
          n147 = Greater Or Equal To 0?(x=w371) -> (x >= 0?=w370:bool)
        }
        n148 = call "Remove Emptys From StrArray.vi"("Array In"=w362) -> ("Array Out"=w358:string[])  [unwired: 10 in]
        n149 = property on="History" class="LstBox (strict)"("Item Names"=w358) -> ()  [unwired: 2 in, 2 out]
      }
    }
  }
